vi "Config_Wifi.vi"() -> ()   [LabVIEW 2025]
doc: "Configura las credenciales de WIFI que se usaran o resetea al firmware base para usar la ESP en modo OFFLINE"
panel:
  in  "Boolean":bool
  in  "RESET":bool
  out "error out":errorcluster
  in  "stop":bool
  in  "OK Button":bool
  in  "Contraseña":string
  in  "SSID":string
  # "Configura tu red para utilizar la ESP32 con capacidades IOT"
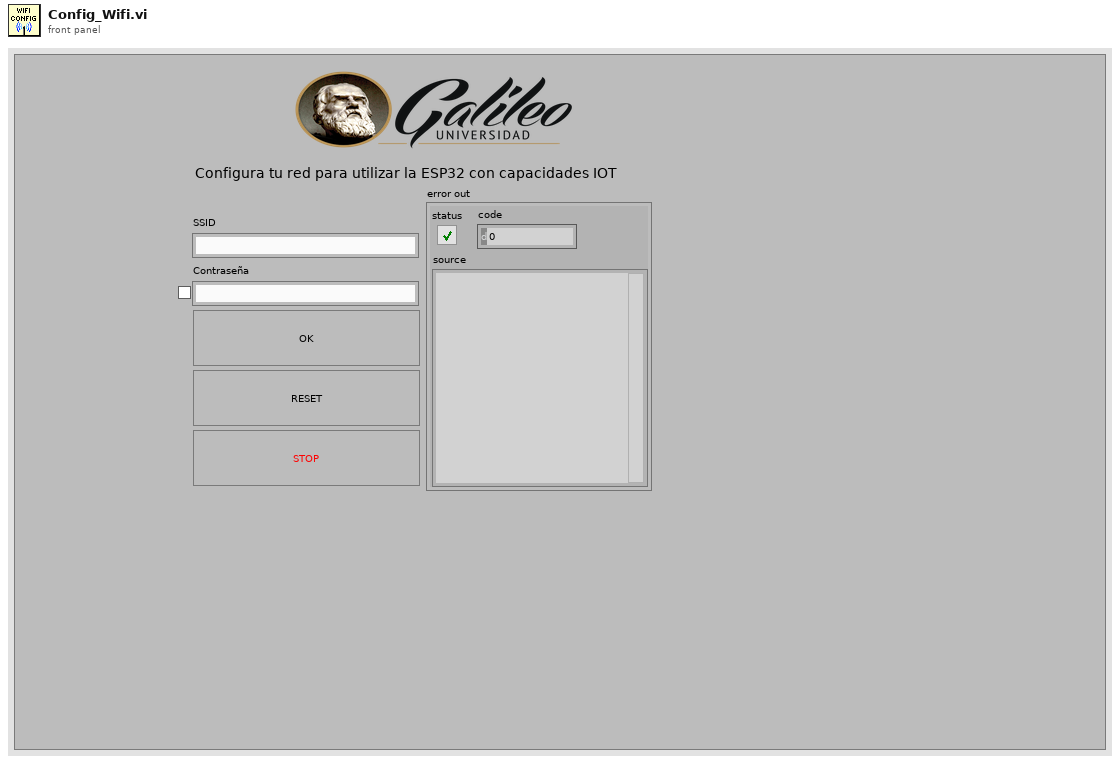
[diagram p1: front panel]
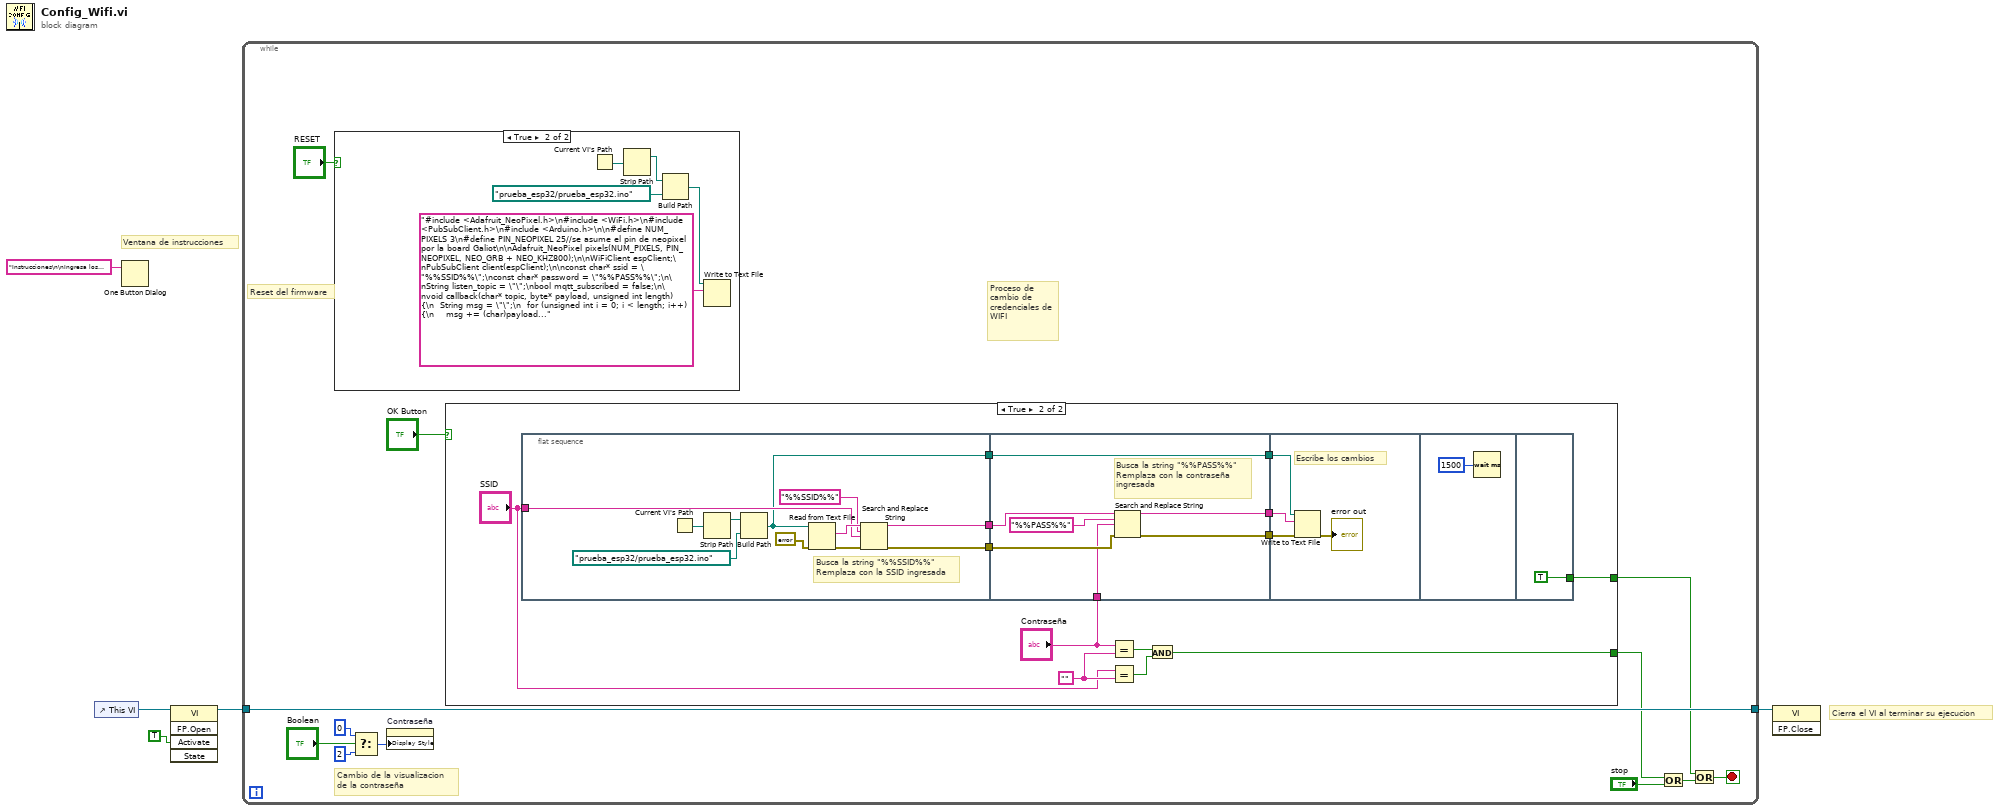
[diagram p0: block diagram]
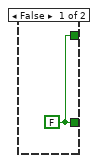
[diagram p3: hidden frame]
diagram:
  # "Cierra el VI al terminar su ejecucion"
  # "Ventana de instrucciones"
  n1 = control-ref of="This VI"() -> (w5:refnum<vi>)
  n2 = One Button Dialog(message="Instrucciones\n\nIngresa los datos de la red a la que te \nquieres conectar.\nIngresa la SSID y su contraseña\nY luego presiona el boton \"OK\" \nSino deseas usar la ESP32 con funciones IOT simplemente presiona el boton \"STOP\" \nPara reestablecer el firmware a su version offline presiona \"RESET\"\n(No se almacenan tus credenciales)") -> ()  [unwired: 1 in, 1 out]
  n3 = invoke class="VI" method="FP.Open"(reference=w5, "Activate"=TRUE ("Activate?")) -> (reference out=w3:refnum<vi>)  [unwired: 3 in, 4 out]
  n4 = while {
    tunnel: w3 -> [w16]
    tunnel: [w16] -> w2
    stop <- w11 stop-if-true
    # "Reset del firmware"
    # "Cambio de la visualizacion\nde la contraseña"
    # "Proceso de cambio de credenciales de WIFI"
    n5 = case shown="True" "RESET" {
      frame False {
      }
      frame True {
        n6 = Current VI's Path() -> (path=w20:path)
        n7 = Strip Path(path=w20) -> (stripped path=w21:path)  [unwired: 1 out]
        n8 = Build Path(base path=w21, name or relative path=path "prueba_esp32/prueba_esp32.ino") -> (appended path=w18:path)
        n9 = Write to Text File(file (use dialog)=w18, text="#include <Adafruit_NeoPixel.h>\n#include <WiFi.h>\n#include <PubSubClient.h>\n#include <Arduino.h>\n\n#define NUM_PIXELS 3\n#define PIN_NEOPIXEL 25//se asume el pin de neopixel por la board Galiot\n\nAdafruit_NeoPixel pixels(NUM_PIXELS, PIN_NEOPIXEL, NEO_GRB + NEO_KHZ800);\n\nWiFiClient espClient;\nPubSubClient client(espClient);\n\nconst char* ssid = \"%%SSID%%\";\nconst char* password = \"%%PASS%%\";\n\nString listen_topic = \"\";\nbool mqtt_subscribed = false;\n\nvoid callback(char* topic, byte* payload, unsigned int length) {\n  String msg = \"\";\n  for (unsigned int i = 0; i < length; i++) {\n    msg += (char)payload[i];\n  }\n  Serial.print(topic);\n  Serial.print(\":\");\n  Serial.println(msg);\n}\n\nvoid setup() {\n  Serial.begin(115200);\n\n  WiFi.begin(ssid, password);\n  unsigned long start = millis();\n  while (WiFi.status() != WL_CONNECTED && millis() - start < 5000) {// intebta conectar sino funciona deja el modo offline\n    delay(500);\n  }\n\n  if (WiFi.status() == WL_CONNECTED) {\n    client.setCallback(callback);\n  } \n\n  pixels.begin();\n  pixels.show();\n}\n\nvoid loop() {\n  static String line = \"\";\n\n  if (Serial.available()) {\n    char peekChar = Serial.peek();\n    if (peekChar == 'A' || peekChar == 'B') {\n      while (Serial.available()) {\n        char c = Serial.read();\n        if (c == '\\n') break;\n        line += c;\n      }\n\n      char tipo = line.charAt(0);\n      line.remove(0, 1);\n      line.trim();\n      int sep = line.indexOf(' ');\n      if (sep > 0) {\n        String ipStr = line.substring(0, sep);\n        String second = line.substring(sep + 1);\n\n        IPAddress brokerIP;\n        if (!brokerIP.fromString(ipStr)) {\n          line = \"\";\n          return;\n        }\n\n        client.setServer(brokerIP, 1883);\n        if (!client.connected()) {\n          if (!client.connect(\"esp32_client\")) {\n            line = \"\";\n            return;\n          }\n        }\n\n        if (tipo == 'A') { // A<ip> <topic> <msg>\n          int sep2 = second.indexOf(' ');\n          if (sep2 > 0) {\n            String topic = second.substring(0, sep2);\n            String msg = second.substring(sep2 + 1);\n            bool ok = client.publish(topic.c_str(), msg.c_str());\n            Serial.write(ok ? 'A' : 'X');\n          }\n        } else if (tipo == 'B') { // B<ip> <topic>\n          listen_topic = second;\n          mqtt_subscribed = client.subscribe(listen_topic.c_str());\n        }\n      }\n\n      line = \"\";\n      return;\n    }\n  }\n\n  if (mqtt_subscribed && client.connected()) {\n    client.loop();\n  }\n\n  if (Serial.available() > 0) {\n    byte instruccion = Serial.read();\n\n    switch (instruccion) {\n      case 0x01: {\n        while (Serial.available() < 2);\n        byte pin = Serial.read();\n        byte val = Serial.read();\n        pinMode(pin, OUTPUT);\n        digitalWrite(pin, val == 0 ? LOW : HIGH);\n        Serial.write('A');\n        break;\n      }\n\n      case 0x02: {\n        while (Serial.available() < 2);\n        byte pin = Serial.read();\n        byte dummy = Serial.read();\n        pinMode(pin, INPUT);\n        byte lectura = digitalRead(pin);\n        Serial.write(lectura ? '1' : '0');\n        break;\n      }\n\n      case 0x03: {\n        while (Serial.available() < 3);\n        byte r = Serial.read();\n        byte g = Serial.read();\n        byte b = Serial.read();\n        for (int i = 0; i < NUM_PIXELS; i++) {\n          pixels.setPixelColor(i, pixels.Color(r, g, b));\n        }\n        pixels.show();\n        Serial.write('A');\n        break;\n      }\n\n      case 0x04: {\n        while (Serial.available() < 4);\n        byte neo = Serial.read();\n        byte r = Serial.read();\n        byte g = Serial.read();\n        byte b = Serial.read();\n        if (neo < NUM_PIXELS) {\n          pixels.setPixelColor(neo, pixels.Color(r, g, b));\n          pixels.show();\n          Serial.write('A');\n        } else {\n          Serial.write('X');\n        }\n        break;\n      }\n\n      case 0x05: {\n        while (Serial.available() < 1);\n        byte pin = Serial.read();\n        int val = analogRead(pin);  // lectura ADC (0–4095)\n        Serial.write(highByte(val));  // Enviamos MSB\n        Serial.write(lowByte(val));   // Enviamos LSB\n        break;\n      }\n\n      case 0x06: {\n        while (Serial.available() < 2);\n        byte pin = Serial.read();\n        byte val = Serial.read();\n        if (pin == 25 || pin == 26) {\n          dacWrite(pin, val);\n          Serial.write('A');\n        } else {\n          Serial.write('X');\n        }\n        break;\n      }\n\n      case 0x07: {\n        while (Serial.available() < 2);\n        byte pin = Serial.read();\n        byte duty = Serial.read(); // 0–255\n\n        ledcAttachChannel(pin, 1000, 8,0);\n        ledcWrite(pin, duty);\n        Serial.write('A');\n        break;\n      }\n\n      case 0xF0: {\n        Serial.write('A');\n        break;\n      }\n\n      case 0xF1: {\n        Serial.write(WiFi.status() == WL_CONNECTED ? 'A' : 'X');//conectado o no\n        break;\n      }\n\n      case 0xF2: {\n        if (mqtt_subscribed && client.connected()) {\n          client.unsubscribe(listen_topic.c_str());\n          mqtt_subscribed = false;\n          listen_topic = \"\";\n        }\n        break;\n      }\n\n      default:\n        //Serial.write('X');\n        break;\n    }\n  }\n}\n") -> ()  [unwired: 2 in, 3 out]
      }
    }
    n10 = Select(t=0, s="Boolean", f=2) -> (s? t:f=w6:i32)
    n11 = property on="Contraseña" class="Str"("Display Style"=w6) -> ()  [unwired: 2 in, 2 out]
    n12 = case shown="True" "OK Button" {
      tunnel: [w23 w33] -> w14
      tunnel: [w23 w24] -> w12
      frame False {
        w23 = FALSE
      }
      frame True {
        w36 = ""
        n13 = flat-sequence {
          tunnel: "SSID" -> [w44]
          tunnel: [w37] -> w31
          tunnel: [w42] -> w30
          tunnel: [w41] -> w28
          tunnel: w31 -> [w48]
          tunnel: w30 -> [w54]
          tunnel: [w53] -> w29
          tunnel: w28 -> [w52]
          tunnel: "Contraseña" -> [w50]
          tunnel: [w49] -> w26
          tunnel: [w48] -> w25
          tunnel: w29 -> [w57]
          tunnel: w26 -> [w55]
          tunnel: w25 -> [w58]
          tunnel: [TRUE] -> w24
          frame #0 {
            # "Busca la string \"%%SSID%%\"\nRemplaza con la SSID ingresada"
            n14 = Current VI's Path() -> (path=w39:path)
            n15 = Strip Path(path=w39) -> (stripped path=w40:path)  [unwired: 1 out]
            n16 = Build Path(base path=w40, name or relative path=path "prueba_esp32/prueba_esp32.ino") -> (appended path=w37:path)
            n17 = Read from Text File(file (use dialog)=w37, error in=errorcluster {"status"=FALSE, "code"=0, "source"=""}) -> (text=w46:string, error out=w43:errorcluster)  [unwired: 2 in, 2 out]
            n18 = Search and Replace String(input string=w46, search string="%%SSID%%", replace string=w44, error in=w43) -> (result string=w41:string, error out=w42:errorcluster)  [unwired: 4 in, 2 out]
          }
          frame #1 {
            # "Busca la string \"%%PASS%%\"\nRemplaza con la contraseña \ningresada"
            n19 = Search and Replace String(input string=w52, search string="%%PASS%%", replace string=w50, error in=w54) -> (result string=w49:string, error out=w53:errorcluster)  [unwired: 4 in, 2 out]
          }
          frame #2 {
            # "Escribe los cambios"
            n20 = Write to Text File(file (use dialog)=w58, text=w55, error in=w57) -> (error out=→"error out":errorcluster)  [unwired: 1 in, 2 out]
          }
          frame #3 {
            n21 = Wait (ms)(milliseconds to wait=u32 1500) -> ()  [unwired: 1 out]
          }
          frame #4 {
          }
        }
        n22 = Equal?(x="Contraseña", y=w36) -> (x = y?=w35:bool)
        n23 = Equal?(x="SSID", y=w36) -> (x = y?=w34:bool)
        n24 = And(x=w35, y=w34) -> (x .and. y?=w33:bool)
      }
    }
    n25 = Or(x=w14, y="stop") -> (x .or. y?=w13:bool)
    n26 = Or(x=w12, y=w13) -> (x .or. y?=w11:bool)
  }
  n27 = invoke class="VI" method="FP.Close"(reference=w2) -> ()  [unwired: 2 in, 3 out]
